vi "Report-Test Details.vi"(7 "Report-Test details":refnum<vi>, 8 "error in (no error)":errorcluster, 11 "all rows":string[][](array[string])) -> (0 "error out":errorcluster)   [LabVIEW 2017]
uses:
  <vilib>/Utility/miscctls.llb/LVDateTimeRec.ctl
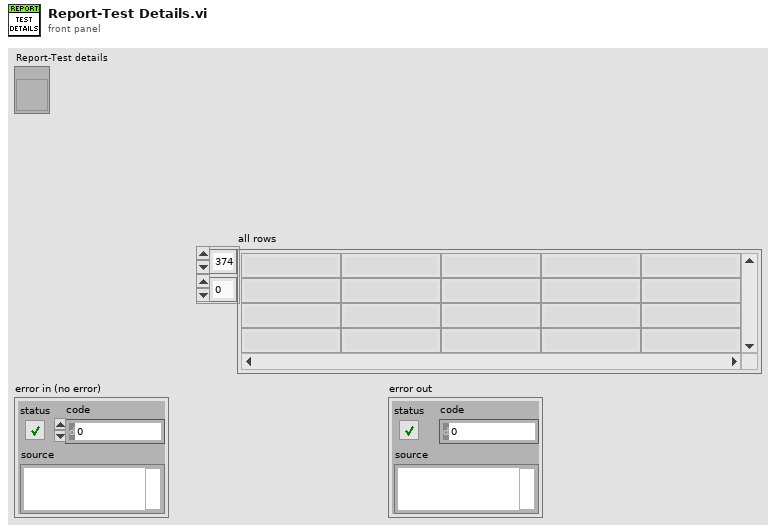
[diagram p1: front panel]
types:
  T1 = typedef "LVDateTimeRec.ctl" = cluster{"fractional second":dbl, "second":i32, "minute":i32, "hour":i32, "day of month":i32, "month":i32, "year":i32, "day of week":i32, "day of year":i32, "DST":i32}
  T2 = cluster{"Date :":string, "Test Start Time: ":string, "Test Stop Time :":string, "Furnace :":string, "Flow :":string, "ID :":string, "Material : ":string, "Angle : ":string, "ID Status :":string}
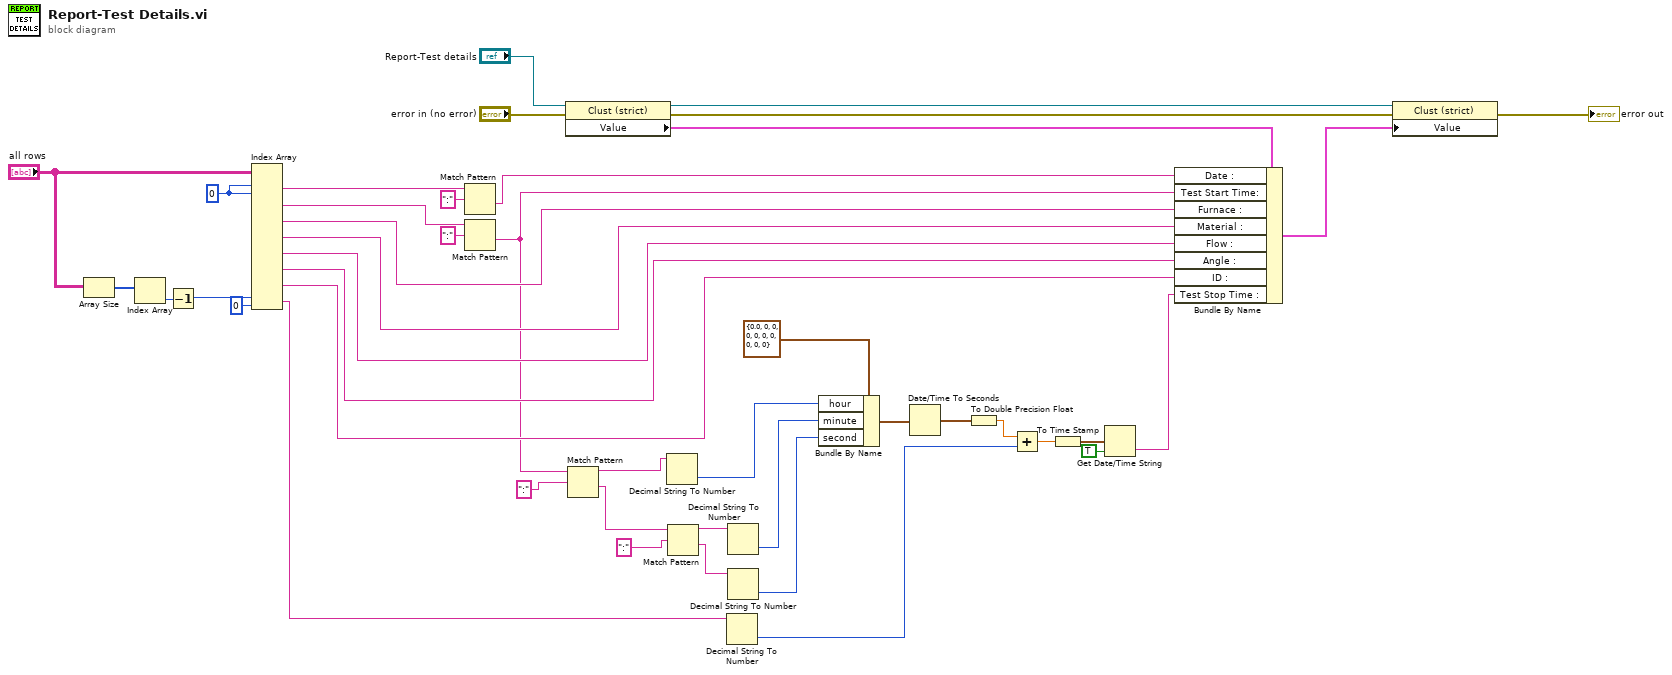
[diagram p0: block diagram]
diagram:
  w43 = 0 ("disabled index (col)")
  n1 = Array Size(array="all rows") -> (size(s)=w29:i32[])
  n2 = Index Array(array=w29) -> (element=w28:i32)  [unwired: 1 in]
  n3 = Decrement(x=w28) -> (x-1=w27:i32)
  n4 = Index Array(array="all rows", index (row) #1=w43, index (col) #1=w43, index (row) #8=w27, index (col) #8=0 ("disabled index (col)")) -> (element #1=w40:string, element #2=w36:string, element #3=w35:string, element #4=w34:string, element #5=w33:string, element #6=w32:string, element #7=w31:string, element #8=w11:string)  [unwired: 12 in]
  n5 = Match Pattern(string=w40, regular expression=":") -> (after substring=w38:string)  [unwired: 1 in, 3 out]
  n6 = Match Pattern(string=w36, regular expression=":") -> (after substring=w23:string)  [unwired: 1 in, 3 out]
  n7 = property class="Clust (strict)"(reference="Report-Test details", error in="error in (no error)") -> (reference out=w4:refnum<vi>, error out=w3:errorcluster, "Value"=w41:T2)
  n8 = Match Pattern(string=w23, regular expression=":") -> (before substring=w21:string, after substring=w19:string)  [unwired: 1 in, 2 out]
  n9 = Decimal String To Number(string=w21) -> (number=w20:i32)  [unwired: 2 in, 1 out]
  n10 = Match Pattern(string=w19, regular expression=":") -> (before substring=w17:string, after substring=w15:string)  [unwired: 1 in, 2 out]
  n11 = Decimal String To Number(string=w11) -> (number=w10:i32)  [unwired: 2 in, 1 out]
  n12 = Decimal String To Number(string=w17) -> (number=w16:i32)  [unwired: 2 in, 1 out]
  n13 = Decimal String To Number(string=w15) -> (number=w14:i32)  [unwired: 2 in, 1 out]
  n14 = Bundle By Name(cluster=T1 {"fractional second"=0.0, "second"=0, "minute"=0, "hour"=0, "day of month"=0, "month"=0, "year"=0, "day of week"=0, "day of year"=0, "DST"=0} ("date time rec"), "hour"=w20, "minute"=w16, "second"=w14) -> (w24:T1)
  n15 = Date/Time To Seconds(2:w24) -> (0:w13:timestamp)  [unwired: 1 in]
  n16 = To Double Precision Float(number=w13) -> (double precision float=w12:dbl)
  n17 = Add(x=w12, y=w10) -> (x+y=w9:dbl)
  n18 = To Time Stamp(1:w9) -> (0:w8:timestamp)
  n19 = Get Date/Time String(seconds (now)=w8, want seconds? (F)=TRUE) -> (time string=w6:string)  [unwired: 1 in, 1 out]
  n20 = Bundle By Name(cluster=w41, "Date :"=w38, "Test Start Time:"=w23, "Furnace :"=w35, "Material :"=w34, "Flow :"=w33, "Angle :"=w32, "ID :"=w31, "Test Stop Time :"=w6) -> (w1:T2)
  n21 = property class="Clust (strict)"(reference=w4, error in=w3, "Value"=w1) -> (error out=→"error out":errorcluster)  [unwired: 1 out]
